vi "Dispose Kinect.vi"(8 "error in (no error)":errorcluster, 11 "input cluster":T1) -> (0 "error out":errorcluster)   [LabVIEW 2011]
uses:
  <vilib>/vision/Image Controls.llb/IMAQ Image.ctl
  Microsoft.Kinect
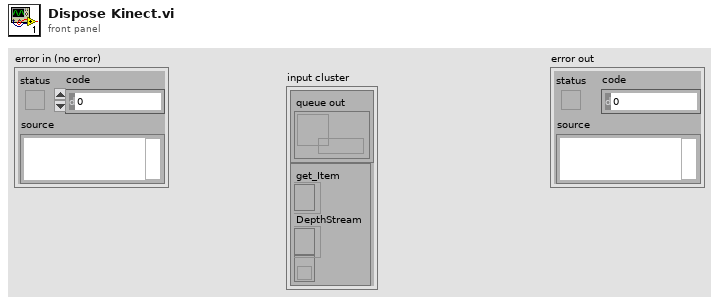
[diagram p1: front panel]
types:
  T1 = cluster{cluster{"queue out":refnum<queue>}, cluster{"get_Item":refnum<k24>, "DepthStream":refnum<k24>, "Event Callback":refnum<k27>}}
  T2 = cluster{"get_Item":refnum<k24>, "DepthStream":refnum<k24>, "Event Callback":refnum<k27>}
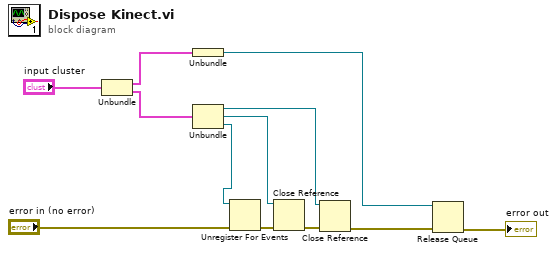
[diagram p0: block diagram]
diagram:
  n1 = Unbundle("input cluster") -> (w12:cluster{"queue out":refnum<queue>}, w11:T2)
  n2 = Unbundle(w12) -> ("queue out"=w9:refnum<queue>)
  n3 = Unbundle(w11) -> ("get_Item"=w8:refnum<k24>, "DepthStream"=w5:refnum<k24>, "Event Callback"=w3:refnum<k27>)
  n4 = Unregister For Events(event registration refnum=w3, error in="error in (no error)") -> (error out=w4:errorcluster)
  n5 = Close Reference(reference=w5, error in (no error)=w4) -> (error out=w6:errorcluster)
  n6 = Close Reference(reference=w8, error in (no error)=w6) -> (error out=w7:errorcluster)
  n7 = Release Queue(queue=w9, error in (no error)=w7) -> (error out=→"error out":errorcluster)  [unwired: 1 in, 2 out]
